vi "VI Example.vi"(8 "error in (no error)":errorcluster, 10 "Data (Dictionary)":T1[](array[typedef])=[{"key"="time", "value"=variant(dbl[] array[87118 elements])}, {"key"="temp", "value"=variant(dbl[] array[87118 elements])}, {"key"="Bfield", "value"=variant(dbl[] array[87118 elements])}, {"key"="X0", "value"=variant(dbl[] array[87118 elements])}, {"key"="Y0", "value"=variant(dbl[] array[87118 elements])}, {"key"="X1", "value"=variant(dbl[] array[87118 elements])}, {"key"="Y1", "value"=variant(dbl[] array[87118 elements])}, {"key"="X2", "value"=variant(dbl[] array[87118 elements])}, {"key"="Y2", "value"=variant(dbl[] array[87118 elements])}, {"key"="X3", "value"=variant(dbl[] array[87118 elements])}, {"key"="Y3", "value"=variant(dbl[] array[87118 elements])}, {"key"="X4", "value"=variant(dbl[] array[87118 elements])}, {"key"="Y4", "value"=variant(dbl[] array[87118 elements])}, {"key"="X5", "value"=variant(dbl[] array[87118 elements])}, {"key"="Y5", "value"=variant(dbl[] array[87118 elements])}, {"key"="X6", "value"=variant(dbl[] array[87118 elements])}, {"key"="Y6", "value"=variant(dbl[] array[87118 elements])}, {"key"="X7", "value"=variant(dbl[] array[87118 elements])}, {"key"="Y7", "value"=variant(dbl[] array[87118 elements])}], 11 "Path":path) -> (0 "error out":errorcluster, 3 "saved file":path=path "C:/")   [LabVIEW 2019]
uses:
  LV-Data/Typedefs/Dictionary--cluster.ctl
  LV-Data/LV-Data.lvclass
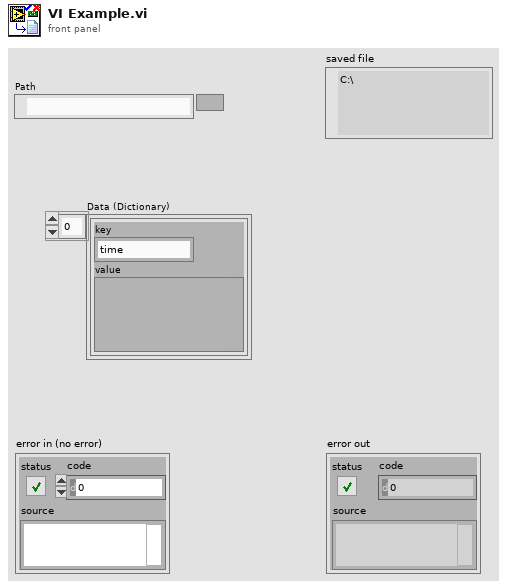
[diagram p1: front panel]
types:
  T1 = typedef "LV-Data.lvclass/Dictionary--cluster.ctl" = cluster{"key":string, "value":variant}
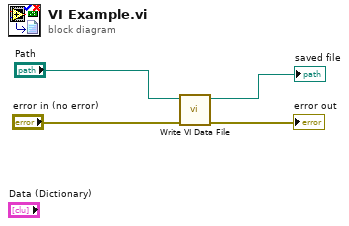
[diagram p0: block diagram]
diagram:
  n1 = call "Write VI Data File.vi"("error in"="error in (no error)", "Path"="Path") -> ("error out"=→"error out":errorcluster, "saved file"=→"saved file":path)  [unwired: 8 in]
